vi "Export IO.vi"(8 "error in (no error)":errorcluster, 10 "GUID":string, 11 "Section Ref in":T5 format="%.0x") -> (0 "error out":errorcluster, 1 "IO":T1 {"Resp"."Signals"."Byte Order" items=["Little Endian", "Big Endian"]; "Resp"."Signals"."Data Type" items=["Signed", "Unsigned", "IEEE Float"]; "Cmd"."Signals"."Byte Order" items=["Little Endian", "Big Endian"]; "Cmd"."Signals"."Data Type" items=["Signed", "Unsigned", "IEEE Float"]}, 2 "IO":T6 {"Resp"."Signal Refs" format="%.0x"; "Cmd"."Signal Refs" format="%.0x"}, 3 "Section Ref out":T5 format="%.0x")   [LabVIEW 2015, in "Diagnostics Addon System Explorer.lvlib"]
uses:
  Diagnostics Addon System Explorer.lvlib
  <vilib>/NI Veristand/Custom Device API/Custom Device Item Ref.ctl
  Types/IO VS References.ctl
  Types/Frame Signal VS References.ctl
  Types/Common IOs.ctl
  Shared/Types/Common Frame Parameters.ctl
  Shared/Types/MessageType Selector.ctl
  Shared/Types/Signal Parameters.ctl
  Types/FG Action.ctl
  Signal Parameters FG.vi
  <vilib>/NI Veristand/Custom Device API/NI VeriStand - Get Custom Device Channel Data.vi
  <vilib>/NI Veristand/Custom Device API/NI VeriStand - Get Item Description.vi
  <vilib>/NI Veristand/Custom Device API/NI VeriStand - Get Item Property.vi
  <vilib>/NI Veristand/Custom Device API/Get Item Property (String).vi
  <vilib>/NI Veristand/Custom Device API/Get Item Property (Double).vi
  <vilib>/NI Veristand/Custom Device API/Get Item Property (U32).vi
  <vilib>/NI Veristand/Custom Device API/NI VeriStand - Set Item Property.vi
  <vilib>/NI Veristand/Custom Device API/Set Item Property (String).vi
  <vilib>/NI Veristand/Custom Device API/Set Item Property (Double).vi
  <vilib>/NI Veristand/Custom Device API/Set Item Property (U32).vi
  Shared/SubVIs/GUID Lookup.vi
  <vilib>/NI Veristand/Custom Device Tools/Custom Device Utility Library/NI VeriStand - Search for Item by GUID.vi
  <vilib>/NI Veristand/Custom Device Tools/Custom Device Utility Library/Custom Device Utility Library.lvlib
  <vilib>/NI Veristand/Custom Device API/Custom Device API.lvlib
  Shared/Diagnostics Addon Shared.lvlib
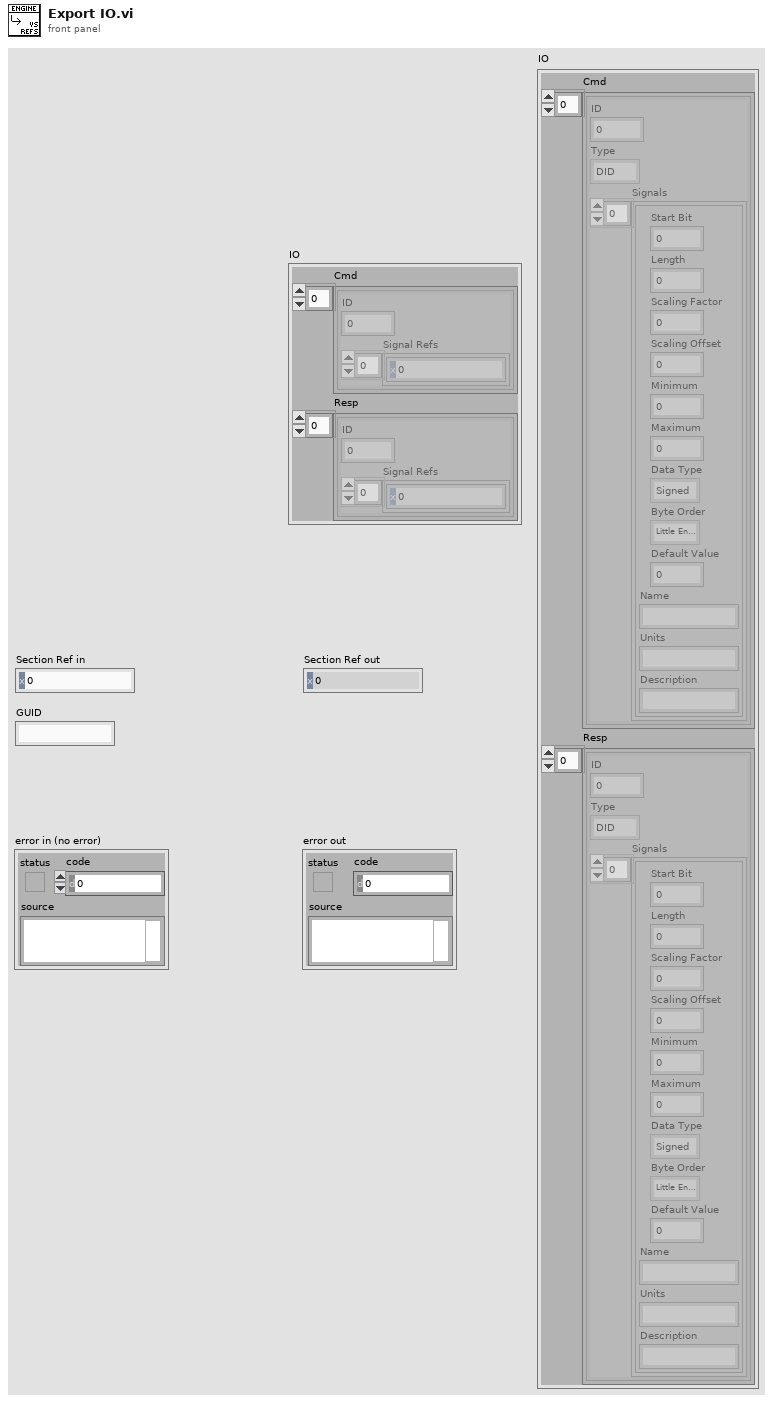
[diagram p1: front panel]
types:
  T1 = typedef "Diagnostics Addon System Explorer.lvlib/Common IOs.ctl" = cluster{"Cmd":T2[], "Resp":T2[]}
  T2 = typedef "Diagnostics Addon Shared.lvlib/Common Frame Parameters.ctl" = cluster{"ID":u32, "Type":T3, "Signals":T4[]}
  T3 = typedef "Diagnostics Addon Shared.lvlib/MessageType Selector.ctl" = enum16{"DID", "CDID", "PID", "CPID", "Write Memory", "Read Memory", "DTC Control", "IO Cmd", "IO Resp", "Routine Start Cmd", "Routine Start Resp", "Routine Status Cmd", "Routine Status Resp", "Routine Stop Cmd", "Routine Stop Resp"}
  T4 = typedef "Diagnostics Addon Shared.lvlib/Signal Parameters.ctl" = cluster{"Start Bit":u8, "Length":u8, "Scaling Factor":dbl, "Scaling Offset":dbl, "Minimum":dbl, "Maximum":dbl, "Data Type":u32, "Byte Order":u32, "Default Value":dbl, "Name":string, "Units":string, "Description":string}
  T5 = typedef "Custom Device API.lvlib/Custom Device Item Ref.ctl" = u64
  T6 = typedef "Diagnostics Addon System Explorer.lvlib/IO VS References.ctl" = cluster{"Cmd":T7[], "Resp":T7[]}
  T7 = typedef "Diagnostics Addon System Explorer.lvlib/Frame Signal VS References.ctl" = cluster{"ID":u32, "Signal Refs":T5[]}
  T8 = typedef "Diagnostics Addon System Explorer.lvlib/FG Action.ctl" = enum16{"Get", "Set"}
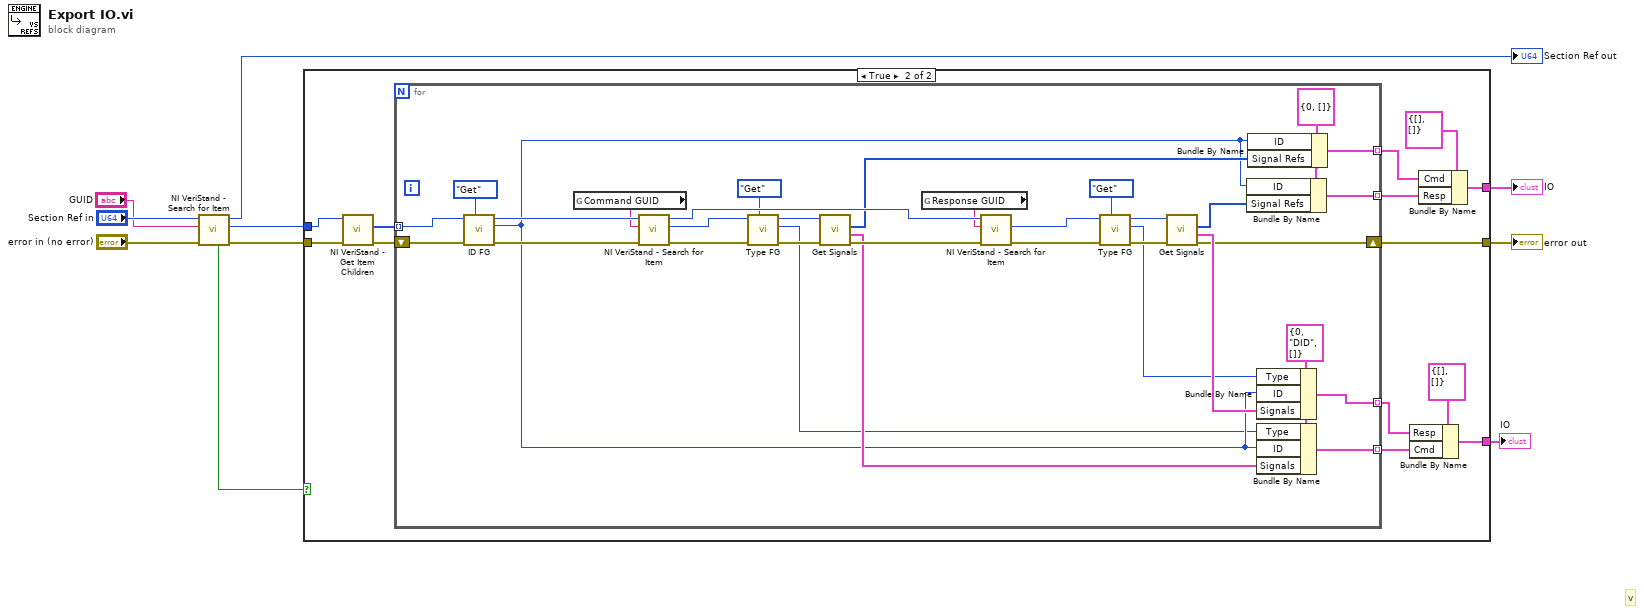
[diagram p0: block diagram]
diagram:
  # "v"
  n1 = call-poly <vilib>:"NI VeriStand - Search for Item.vi"("error in"="error in (no error)", "Item GUID"="GUID", "Section Ref in"="Section Ref in") -> ("error out"=w4:errorcluster, "Item Ref"=w5:T5, "Section Ref out"=→"Section Ref out":T5, "Found"=w2:bool)  [unwired: 5 in]
  n2 = case shown="True" w2 {
    tunnel: [w11 w24] -> w9
    tunnel: [_ w12] -> w8
    tunnel: w5 -> [_ w21]
    tunnel: w4 -> [w11 w20]
    tunnel: [_ w18] -> w1
    frame False {
    }
    frame True {
      n3 = call <vilib>:"NI VeriStand - Get Item Children.vi"("error in (no error)"=w20, "Item Ref in"=w21) -> ("error out"=w22:errorcluster, "Child Refs"=w23:T5[])  [unwired: 6 in, 2 out]
      n4 = for {
        shift-right: [w45] -> w24
        shift-left: w22 -> [w52]
        tunnel: w23 -> [w51] mode=indexing
        tunnel: [w44] -> w16 mode=indexing
        tunnel: [w43] -> w19 mode=indexing
        tunnel: [w38] -> w14 mode=indexing
        tunnel: [w37] -> w13 mode=indexing
        w41 = T7 {"ID"=0, "Signal Refs"=[]} ("Cmd")
        w57 = T2 {"ID"=0, "Type"=enum."DID", "Signals"=[]} ("PID In")
        n5 = call "ID FG.vi"("Action"=FG_Action."Get", "error in (no error)"=w52, "Device Item Ref in"=w51) -> ("error out"=w49:errorcluster, "ID"=w40:u32, "Device Item Ref out"=w50:T5)  [unwired: 6 in]
        n6 = global read "GUID Lookup.vi" "Command GUID"() -> (w48:string)
        n7 = call-poly <vilib>:"NI VeriStand - Search for Item.vi"("error in"=w49, "Item GUID"=w48, "Section Ref in"=w50) -> ("error out"=w36:errorcluster, "Item Ref"=w34:T5, "Section Ref out"=w55:T5)  [unwired: 5 in, 1 out]
        n8 = call "Type FG.vi"("Action"=FG_Action."Get", "error in (no error)"=w36, "Device Item Ref in"=w34) -> ("error out"=w35:errorcluster, "Type"=w25:T3, "Device Item Ref out"=w33:T5)  [unwired: 6 in]
        n9 = call "Get Signals.vi"("error in (no error)"=w35, "Device Item Ref out"=w33) -> ("error out"=w56:errorcluster, "Parameters"=w47:T4[], "Child Refs"=w42:T5[])  [unwired: 6 in, 1 out]
        n10 = global read "GUID Lookup.vi" "Response GUID"() -> (w54:string)
        n11 = call-poly <vilib>:"NI VeriStand - Search for Item.vi"("error in"=w56, "Item GUID"=w54, "Section Ref in"=w55) -> ("error out"=w30:errorcluster, "Item Ref"=w28:T5)  [unwired: 5 in, 2 out]
        n12 = call "Type FG.vi"("Action"=FG_Action."Get", "error in (no error)"=w30, "Device Item Ref in"=w28) -> ("error out"=w29:errorcluster, "Type"=w26:T3, "Device Item Ref out"=w27:T5)  [unwired: 6 in]
        n13 = call "Get Signals.vi"("error in (no error)"=w29, "Device Item Ref out"=w27) -> ("error out"=w45:errorcluster, "Parameters"=w46:T4[], "Child Refs"=w39:T5[])  [unwired: 6 in, 1 out]
        n14 = Bundle By Name(cluster=w41, "ID"=w40, "Signal Refs"=w39) -> (w37:T7)
        n15 = Bundle By Name(cluster=w41, "ID"=w40, "Signal Refs"=w42) -> (w38:T7)
        n16 = Bundle By Name(cluster=w57, "Type"=w26, "ID"=w40, "Signals"=w46) -> (w44:T2)
        n17 = Bundle By Name(cluster=w57, "Type"=w25, "ID"=w40, "Signals"=w47) -> (w43:T2)
      }
      n18 = Bundle By Name(cluster=T1 {"Cmd"=[], "Resp"=[]} ("IO"), "Resp"=w16, "Cmd"=w19) -> (w18:T1)
      n19 = Bundle By Name(cluster=T6 {"Cmd"=[], "Resp"=[]} ("IO"), "Cmd"=w14, "Resp"=w13) -> (w12:T6)
    }
  }
  "error out" <- w9
  "IO" <- w8
  "IO" <- w1
